vi "AddCategory.vi"(8 "error in (no error)":errorcluster, 11 "TimeTracker in":refnum<class "TimeTracker.lvclass">) -> (0 "error out":errorcluster, 3 "TimeTracker out":refnum<class "TimeTracker.lvclass">)   [LabVIEW 2016, in "TimeTracker.lvclass"]
uses:
  TimeTracker.lvclass
  TimeTracker.lvclass/TimeTracker.ctl
  Category.ctl
panel:
  in  "Name":string caption="Category Name"
  in  "Cancel":bool
  in  "OK":bool
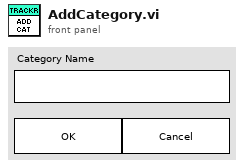
[diagram p1: front panel]
types:
  T1 = typedef "TimeTracker.lvclass/Category.ctl" = cluster{"ID":u32, "Name":string}
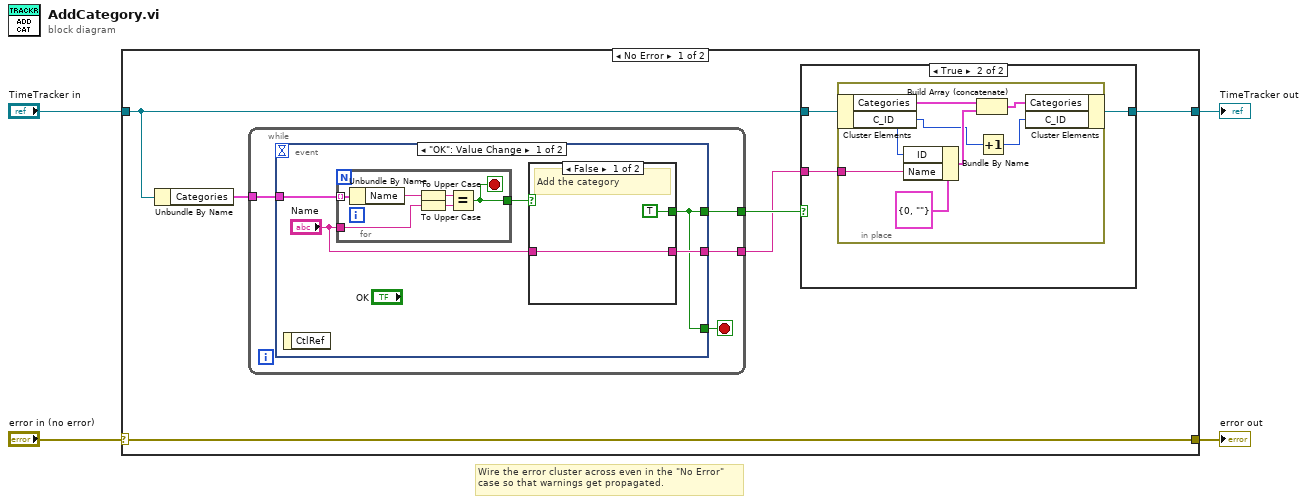
[diagram p0: block diagram]
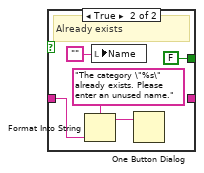
[diagram p3: hidden frame]
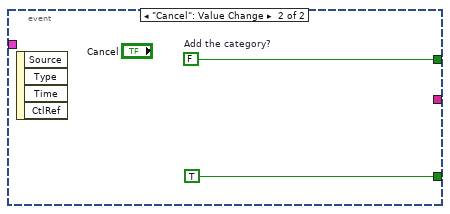
[diagram p4: hidden frame]
diagram:
  # "Wire the error cluster across even in the \"No Error\"\ncase so that warnings get propagated."
  n1 = case shown="No Error" "error in (no error)" {
    selector: "error in (no error)" -> [w10 w47]
    tunnel: [w10 w47] -> w3
    tunnel: [w9 w46] -> w1
    tunnel: "TimeTracker in" -> [w8 w46]
    frame No Error {
      n2 = Unbundle By Name(w8) -> ("Categories"=w7:T1[])
      n3 = while {
        tunnel: w7 -> [w25]
        tunnel: [w23] -> w6
        tunnel: [w22] -> w5
        stop <- w24 stop-if-true
        n4 = event shown="[0] \"OK\": Value Change" {
          selector: _ -> [_ _]
          dyn-events: _ -> [_ _]
          timeout: _ -> [_ _]
          tunnel: w25 -> [w30 _]
          tunnel: [w26 TRUE] -> w24
          tunnel: [w26 w44] -> w23
          tunnel: [w27 _] -> w22
          event "OK": Value Change {
            n5 = event-data() -> ()  [unwired: 1 in, 1 out]
            n6 = for {
              tunnel: w30 -> [w43] mode=indexing
              tunnel: "Name" -> [w41]
              tunnel: [w40] -> w29
              stop <- w40 stop-if-true
              n7 = Unbundle By Name(w43) -> ("Name"=w42:string)
              n8 = To Upper Case(1:w42) -> (0:w39:string)
              n9 = To Upper Case(1:w41) -> (0:w38:string)
              n10 = Equal?(x=w39, y=w38) -> (x = y?=w40:bool)
            }
            n11 = case shown="False" w29 {
              tunnel: "Name" -> [w31 w34]
              tunnel: [w31 _] -> w27
              tunnel: [TRUE FALSE] -> w26
              frame False {
                # "Add the category"
              }
              frame True {
                # "Already exists"
                n12 = Format Into String(format string="The category \"%s\" already exists. Please enter an unused name.", w34) -> (resulting string=w35:string)  [unwired: 2 in, 1 out]
                n13 = local write "Name"("") -> ()
                n14 = One Button Dialog(message=w35) -> ()  [unwired: 1 in, 1 out]
              }
            }
          }
          event "Cancel": Value Change {
            w44 = FALSE  # Add the category?
            n15 = event-data() -> ()  [unwired: 1 in, 4 out]
          }
        }
      }
      n16 = case shown="True" w6 {
        tunnel: [w11 w14] -> w9
        tunnel: w8 -> [w11 w13]
        tunnel: w5 -> [_ w12]
        frame False {
        }
        frame True {
          n17 = in-place {
            in-place-border: w12 -> [w17]
            n18 = in-place-cluster #1(w13) -> ("Categories"=w21:T1[], "C_ID"=w16:u32)
            n19 = Bundle By Name(cluster=T1 {"ID"=0, "Name"=""} ("Category"), "ID"=w16, "Name"=w17) -> (w18:T1)
            n20 = Build Array (concatenate)(w21, w18) -> (w20:T1[])
            n21 = Increment(x=w16) -> (x+1=w15:u32)
            n22 = in-place-cluster #1("Categories"=w20, "C_ID"=w15) -> (w14:refnum<class "TimeTracker.lvclass">)
          }
        }
      }
    }
    frame Error {
    }
  }
  "error out" <- w3
  "TimeTracker out" <- w1
